vi "Query Output State.vi"(8 "error in (no error)":errorcluster, 9 "output state (Constant Voltage)":i32(ring) items=["Constant Voltage"=0, "Constant Current"=1, "Unregulated"=4, "Over Voltage"=2, "Over Current"=3], 10 "channel name (\"CHANNEL1\")":string="CHANNEL1", 11 "CS++DCPwr in":refnum<class "CS++DCPwr.lvclass">) -> (0 "error out":errorcluster, 2 "in state":bool, 3 "CS++DCPwr out":refnum<class "CS++DCPwr.lvclass">)   [LabVIEW 2013, in "CS++DCPwr.lvlib" / "CS++DCPwr.lvclass"]
doc: "This VI returns whether the power supply is in a particular output state.\n\nA constant voltage condition occurs when the output voltage is equal to the value of the IviDCPwr>>Basic Operation>>Voltage Level property and the current is less than or equal to the value of the IviDCPwr>>Basic Operation>>Current Limit property.\n\nA constant current condition occurs when the output current is equal to the value of the IviDCPwr>>Basic Operation>>Current Limit property and the IviDCPwr>>Basic Operation>>Current Limit Behavior property is set to IVIDCPWR_VAL_CURRENT_REGULATE.\n\nAn unregulated condition occurs when the output voltage is less than the value of the IviDCPwr>>Basic Operation>>Voltage Level property and the current is less than the value of the IviDCPwr>>Basic Operation>>Current Limit property.\n\nAn over-voltage condition occurs when the output voltage is equal to or greater than the value of the IviDCPwr>>Basic Operation>>OVP Limit property and the IviDCPwr>>Basic Operation>>OVP Enabled property is set to TRUE.\n\nAn over-current condition occurs when the output current is equal to or greater than the value of the IviDCPwr>>Basic Operation>>Current Limit property and the IviDCPwr>>Basic Operation>>Current Limit Behavior property is set to IVIDCPWR_VAL_CURRENT_TRIP. \n\nWhen either an over-voltage condition or an over-current condition occurs, the power supply's output protection disables the output. If the power supply is in an over-voltage or over-current state, it does not produce power until the output protection is reset. The IviDCPwr Reset Output Protection VI resets the output protection. Once the output protection is reset, the power supply resumes generating a power signal."
uses:
  CS++DCPwr.lvclass
  CSPP_Core/Classes/CS++ProcessVariables/ProcessVariable/PV.lvclass
  PV-Enum.ctl
  CS++DCPwr.lvclass/CS++DCPwr.ctl
  CSPP_Core/Classes/CS++ProcessVariables/ProcessVariable/PV.lvclass/PV.ctl
  CSPP_Core/Classes/CS++ProcessVariables/PVConnection/PVConnection.lvclass
  CSPP_Core/Classes/CS++ProcessVariables/ProcessVariable/Write Data.vi
  CSPP_Core/Classes/CS++ProcessVariables/ProcessVariable/Write Timestamp.vi
  CSPP_Core/Classes/CS++ProcessVariables/ProcessVariable/Write Quality.vi
  CSPP_Core/Classes/CS++ProcessVariables/ProcessVariable/Write status.vi
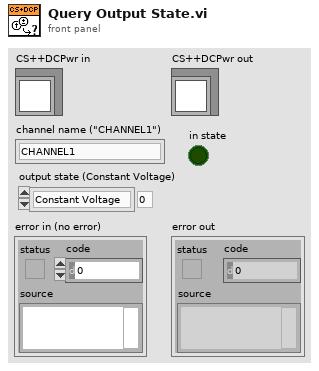
[diagram p1: front panel]
types:
  T1 = typedef "CS++DCPwr.lvlib/CS++DCPwr.lvclass/PV-Enum.ctl" = enum16{"CurrentLimit", "MaxCurrentLimit", "MaxVoltageLevel", "Measure-A", "Measure-V", "OVPLimit", "Range", "TriggerCurrentLimit", "TriggerVoltageLevel", "VoltageLevel", "Behavior", "DesiredOutputState", "RangeType", "TriggerSource", "InState", "OutputEnable", "OVPEnabled"}
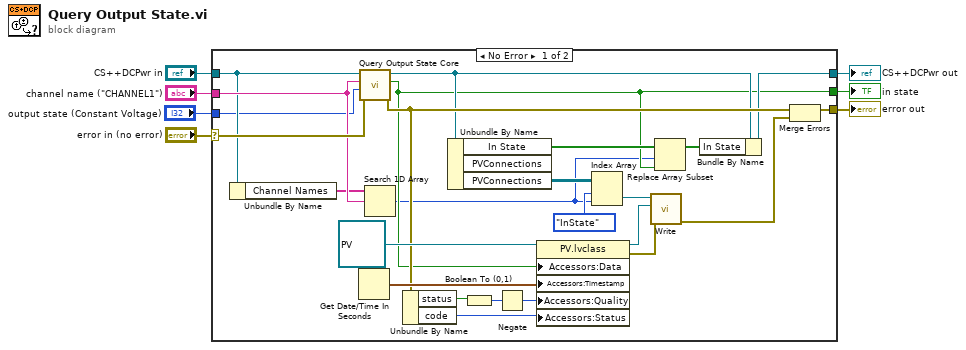
[diagram p0: block diagram]
diagram:
  n1 = case shown="No Error" "error in (no error)" {
    selector: "error in (no error)" -> [w32 w34]
    tunnel: [w25 w34] -> w6
    tunnel: [w16 w33] -> w4
    tunnel: "CS++DCPwr in" -> [w11 w33]
    tunnel: "channel name (\"CHANNEL1\")" -> [w28 _]
    tunnel: [w13 _] -> w2
    tunnel: "output state (Constant Voltage)" -> [w8 _]
    frame No Error {
      n2 = Unbundle By Name(w11) -> ("Channel Names"=w10:string[])
      n3 = Get Date/Time In Seconds() -> (seconds since 1Jan1904=w31:timestamp)
      n4 = call-dynamic "Query Output State Core.vi"("error in (no error)"=w32, "output state (Constant Voltage)"=w8, "channel name (\"CHANNEL1\")"=w28, "CS++DCPwr in"=w11) -> ("error out"=w20:errorcluster, "in state"=w13:bool, "CS++DCPwr out"=w17:refnum<class "CS++DCPwr.lvclass">)  [unwired: 5 in]
      n5 = Search 1D Array(1D array=w10, element=w28) -> (index of element=w9:i32)  [unwired: 1 in]
      n6 = Unbundle By Name(w20) -> ("status"=w24:bool, "code"=w22:i32)
      n7 = Unbundle By Name(w17) -> ("In State"=w19:bool[], "PVConnections"=w27:refnum<class "PVConnection.lvclass">[][])  [unwired: 1 out]
      n8 = Boolean To (0,1)(Boolean=w24) -> (0, 1=w23:i16)
      n9 = Negate(x=w23) -> (-x=w21:i16)
      n10 = property class="PV.lvclass"(reference=refnum<class "PV.lvclass"> refnum ("PV"), "Accessors:Data"=w13, "Accessors:Timestamp"=w31, "Accessors:Quality"=w21, "Accessors:Status"=w22) -> (reference out=w15:refnum<class "PV.lvclass">, error out=w29:errorcluster)  [unwired: 1 in]
      n11 = Index Array(array=w27, index (row)=PV-Enum."InState" ("PV-Enum"), index (col)=w9) -> (element=w26:refnum<class "PVConnection.lvclass">)
      n12 = call-dynamic "Write.vi"("error in (no error)"=w29, "PV"=w15, "PVConnection in"=w26) -> ("error out"=w14:errorcluster)  [unwired: 7 in, 1 out]
      n13 = Replace Array Subset(array=w19, new element=w13, index=w9) -> (w18:bool[])
      n14 = Bundle By Name(cluster=w17, "In State"=w18) -> (w16:refnum<class "CS++DCPwr.lvclass">)
      n15 = Merge Errors(w20, w14) -> (w25:errorcluster)
    }
    frame Error {
    }
  }
  "error out" <- w6
  "CS++DCPwr out" <- w4
  "in state" <- w2
